vi "Queue_Driver.vi"(0 "Queue Name":string, 5 "State":string, 7 "Array of States":string[](array[string]), 11 "Error In":errorcluster, 13 "Queue Operation":T1) -> (4 "Dequeue Element":string, 15 "Error Out":errorcluster)   [LabVIEW 2020]
uses:
  Typedef/Queue_Operations.ctl
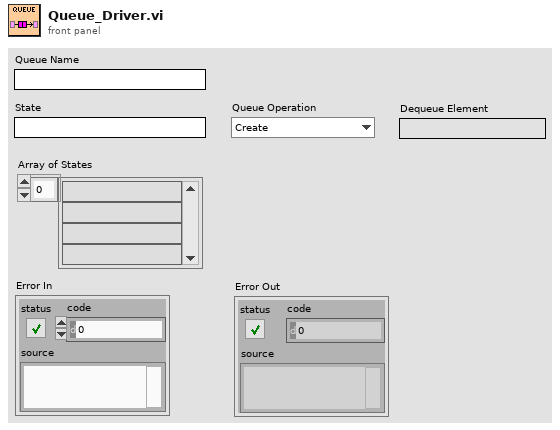
[diagram p1: front panel]
types:
  T1 = typedef "Queue_Operations.ctl" = enum16{"Create", "Enqueue", "Enqueue N", "Dequeue", "Enstack", "Flush", "Release"}
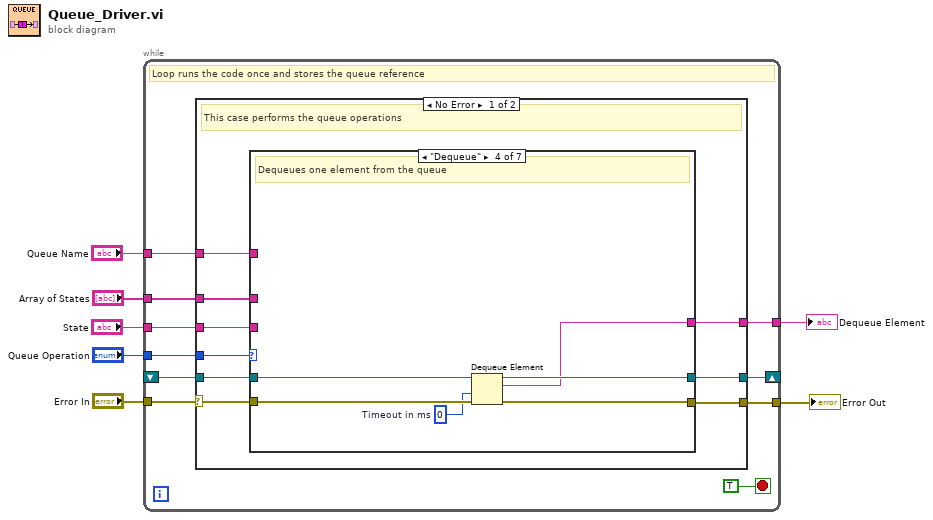
[diagram p0: block diagram]
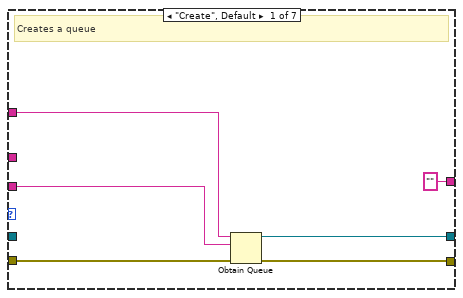
[diagram p2: hidden frame]
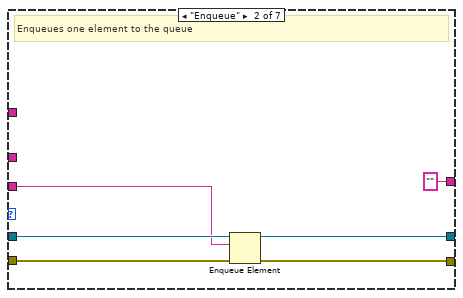
[diagram p3: hidden frame]
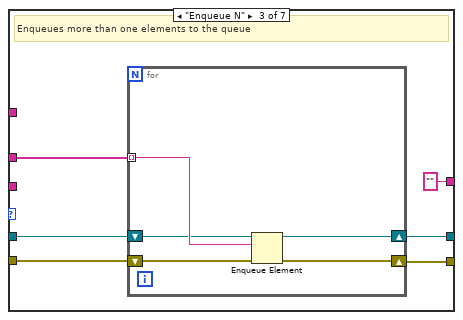
[diagram p4: hidden frame]
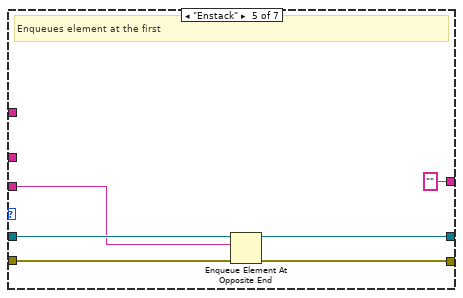
[diagram p5: hidden frame]
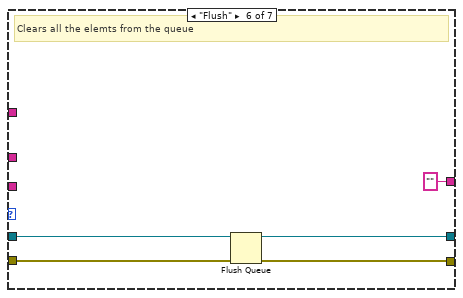
[diagram p6: hidden frame]
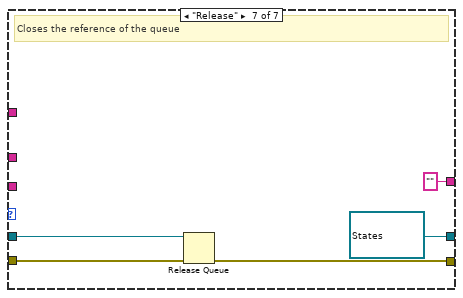
[diagram p7: hidden frame]
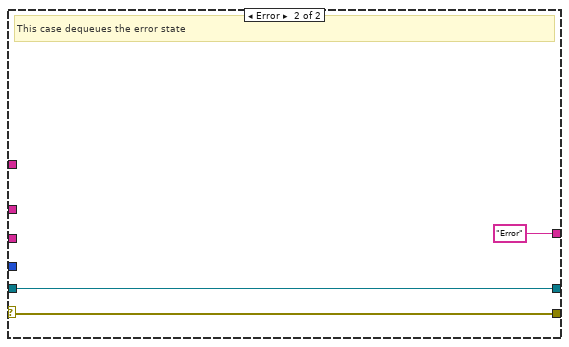
[diagram p8: hidden frame]
diagram:
  n1 = while {
    tunnel: "Error In" -> [w17]
    tunnel: "Queue Operation" -> [w16]
    tunnel: "Queue Name" -> [w15]
    tunnel: "State" -> [w14]
    tunnel: "Array of States" -> [w13]
    shift-right: [w12] -> _
    shift-left: _ -> [w11]
    tunnel: [w10] -> w2
    tunnel: [w8] -> w1
    stop <- TRUE stop-if-true
    # "Loop runs the code once and stores the queue reference"
    n2 = case shown="No Error" w17 {
      selector: w17 -> [w26 w73]
      tunnel: w16 -> [w25 _]
      tunnel: w15 -> [w24 _]
      tunnel: w14 -> [w23 _]
      tunnel: w13 -> [w22 _]
      tunnel: [w21 w74] -> w12
      tunnel: w11 -> [w20 w74]
      tunnel: [w19 w73] -> w10
      tunnel: [w18 "Error" ("Queue Name")] -> w8
      frame No Error {
        # "This case performs the queue operations"
        n3 = case shown="\"Dequeue\"" w25 {
          tunnel: [w31 w37 w43 w54 w60 w65 w70] -> w19
          tunnel: w26 -> [w32 w38 w44 w55 w61 w66 w71]
          tunnel: w24 -> [w30 _ _ _ _ _ _]
          tunnel: w23 -> [w29 w35 _ _ w57 _ _]
          tunnel: w22 -> [_ _ w42 _ _ _ _]
          tunnel: [w28 w34 w40 w53 w58 w63 refnum<queue> refnum ("queue out")] -> w21
          tunnel: w20 -> [_ w36 w41 w52 w59 w64 w69]
          tunnel: ["" ("States") "" ("States") "" ("States") w50 "" ("States") "" ("States") "" ("States")] -> w18
          frame "Create", Default {
            # "Creates a queue"
            n4 = Obtain Queue(name (unnamed)=w30, element data type=w29, error in (no error)=w32) -> (queue out=w28:refnum<queue>, error out=w31:errorcluster)  [unwired: 2 in, 1 out]
          }
          frame "Enqueue" {
            # "Enqueues one element to the queue"
            n5 = Enqueue Element(queue=w36, element=w35, error in (no error)=w38) -> (queue out=w34:refnum<queue>, error out=w37:errorcluster)  [unwired: 1 in, 1 out]
          }
          frame "Enqueue N" {
            # "Enqueues more than one elements to the queue"
            n6 = for {
              shift-right: [w48] -> w43
              shift-left: w44 -> [w49]
              tunnel: w42 -> [w47] mode=indexing
              shift-right: [w45] -> w40
              shift-left: w41 -> [w46]
              n7 = Enqueue Element(queue=w46, element=w47, error in (no error)=w49) -> (queue out=w45:refnum<queue>, error out=w48:errorcluster)  [unwired: 1 in, 1 out]
            }
          }
          frame "Dequeue" {
            w51 = 0  # Timeout in ms
            # "Dequeues one element from the queue"
            n8 = Dequeue Element(queue=w52, timeout in ms (-1)=w51, error in (no error)=w55) -> (queue out=w53:refnum<queue>, element=w50:string, error out=w54:errorcluster)  [unwired: 1 out]
          }
          frame "Enstack" {
            # "Enqueues element at the first"
            n9 = Enqueue Element At Opposite End(queue=w59, element=w57, error in (no error)=w61) -> (queue out=w58:refnum<queue>, error out=w60:errorcluster)  [unwired: 1 in, 1 out]
          }
          frame "Flush" {
            # "Clears all the elemts from the queue"
            n10 = Flush Queue(queue=w64, error in (no error)=w66) -> (queue out=w63:refnum<queue>, error out=w65:errorcluster)  [unwired: 1 out]
          }
          frame "Release" {
            # "Closes the reference of the queue"
            n11 = Release Queue(queue=w69, error in (no error)=w71) -> (error out=w70:errorcluster)  [unwired: 1 in, 2 out]
          }
        }
      }
      frame Error {
        # "This case dequeues the error state"
      }
    }
  }
  "Error Out" <- w2
  "Dequeue Element" <- w1
